vi "GetI_AAAa.vi"(8 "error in (no error)":errorcluster, 11 "reference in":refnum<class "GOOP4_Sub.lvclass">) -> (0 "error out":errorcluster, 2 "InterfaceOut":refnum<class "AAAa.lvclass">, 3 "reference out":refnum<class "GOOP4_Sub.lvclass">)   [LabVIEW 2019, in "GOOP4_Sub.lvclass"]
doc: "Returns an Interaface that this class implements"
uses:
  GOOP4_Sub.lvclass
  AAAa_Interface/AAAa.lvclass
  GOOP4_Sub.lvclass/GOOP4_Sub.ctl
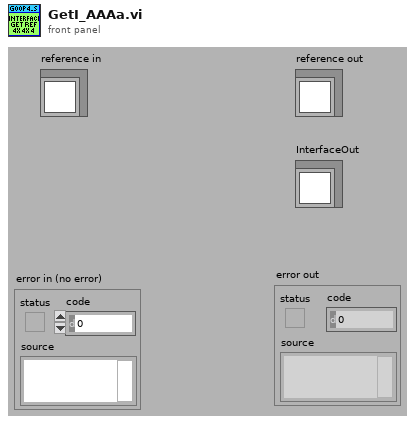
[diagram p1: front panel]
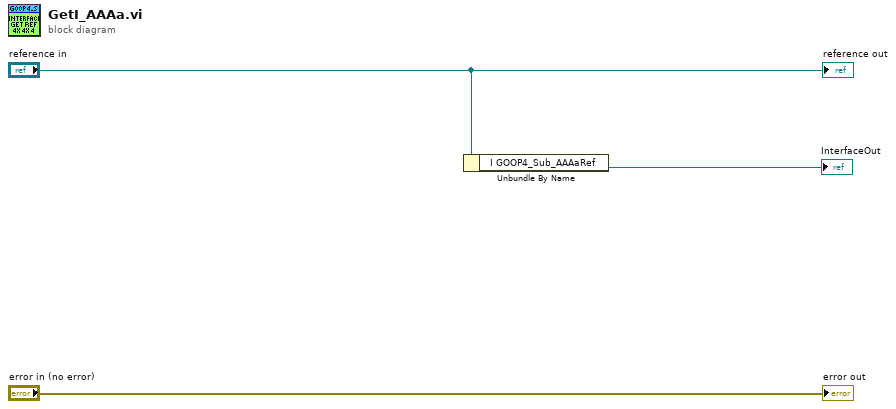
[diagram p0: block diagram]
diagram:
  n1 = Unbundle By Name("reference in") -> ("I GOOP4_Sub_AAAaRef"=→"InterfaceOut":refnum<class "AAAa.lvclass">)
  "error out" <- "error in (no error)"
  "reference out" <- "reference in"
